vi "Gauss-fit_smpl.vi"(5 "parameter bounds":T2, 6 "initial guess":T1, 10 "FF array":dbl[](array[numeric])=[275.0, 9.0, -4.0, 1.0, -14.0, 8.0, 1.0, 17.0, -3.0, 12.0, 6.0, 9.0, -11.0, -4.0, -2.0, 0.0, -2.0, -7.0, 7.0, -2.0, -2.0, -13.0, 2.0, -1.0, -16.0, 3.0, -2.0, -3.0, 2.0, -2.0, 1.0, -1.0, -15.0, -12.0, -11.0, -10.0, -8.0, 13.0, -3.0, 3.0, 10.0, 2.0, -4.0, 2.0, 5.0, 9.0, 20.0, 3.0, -2.0, 9.0, -1.0, 9.0, -8.0, 11.0, 8.0, 19.0, 1.0, -1.0, -1.0, -9.0, -4.0, -5.0, -2.0, -4.0, -16.0, -10.0, -11.0, -12.0, -4.0, -3.0, -10.0, -5.0, -6.0, -8.0, 10.0, 11.0, -9.0, 2.0, 5.0, 6.0, -7.0, 1.0, 2.0, -2.0, -4.0, -10.0, -8.0, 2.0, -3.0, -7.0, 5.0, 5.0, -8.0, 2.0, -3.0, 19.0, -1.0, 9.0, 10.0, 19.0, 10.0, 9.0, 14.0, 8.0, 0.0, 6.0, 5.0, 3.0, -10.0, -7.0, 0.0, -12.0, -21.0, -3.0, -14.0, 5.0, -4.0, 2.0, -2.0, 0.0, -8.0, 12.0, 1.0, -5.0, -10.0, -8.0, -4.0, -12.0, 1.0, -12.0, -7.0, 7.0, 5.0, 7.0, -3.0, 13.0, 16.0, 13.0, -16.0, 25.0, 7.0, -1.0, 1.0, 20.0, 16.0, 7.0, 9.0, 13.0, 7.0, 10.0, 5.0, 6.0, -1.0, -1.0, -2.0, -10.0, -15.0, -8.0, -27.0, -5.0, -7.0, 5.0, 2.0, 15.0, 3.0, 0.0, 8.0, -1.0, 1.0, 3.0, -6.0, 0.0, 3.0, 0.0, -12.0, 7.0, -7.0, -3.0, 3.0, 2.0, 0.0, -12.0, 4.0, -3.0, -7.0, 6.0, -11.0, 6.0, 0.0, -3.0, -4.0, 1.0, 1.0, 4.0, -6.0, 14.0, 3.0, 7.0, 5.0, 4.0, 2.0, 4.0, 13.0, 0.0, 6.0, -12.0, 0.0, 2.0, -9.0, -4.0, 9.0, 11.0, -2.0, 10.0, 1.0, 4.0, 14.0, 3.0, -1.0, 19.0, 12.0, -12.0, 7.0, -14.0, -5.0, 1.0, -1.0, -8.0, -2.0, -7.0, 0.0, -2.0, 5.0, -8.0, -2.0, 14.0, -6.0, 6.0, 5.0, 4.0, 5.0, -3.0, -8.0, -9.0, -15.0, 8.0, -2.0, 3.0, -3.0, 12.0, 4.0, 9.0, 1.0, 10.0, 4.0, 6.0, 0.0, -13.0, -15.0, -8.0, -9.0, -8.0, -6.0, -20.0, -3.0, -6.0, -8.0, 1.0, -7.0, -17.0, -4.0, 2.0, -17.0, 1.0, -2.0, 4.0, 4.0, 14.0, -1.0, 5.0, -1.0, 7.0, -3.0, -2.0, 5.0, -1.0, 8.0, 11.0, 15.0, 3.0, 12.0, 20.0, 5.0, 13.0, 6.0, 22.0, 1.0, 4.0, 7.0, 15.0, 4.0, -1.0, 13.0, 11.0, 6.0, 3.0, 8.0, -2.0, -3.0, 9.0, 15.0, 5.0, 16.0, 5.0, 2.0, 5.0, -5.0, 5.0, -7.0, -8.0, -8.0, -11.0, -13.0, -1.0, -12.0, 6.0, -2.0, 11.0, -2.0, 2.0, -12.0, -10.0, -13.0, -4.0, -13.0, -9.0, 8.0, -5.0, -7.0, -8.0, -8.0, 1.0, -1.0, 4.0, 12.0, 3.0, 8.0, 2.0, 3.0, 6.0, -12.0, 12.0, 5.0, 4.0, 2.0, -10.0, 3.0, -9.0, 8.0, 16.0, -6.0, 7.0, -2.0, 15.0, 7.0, 12.0, -1.0, 19.0, 5.0, -17.0, -8.0, -1.0, -15.0, 2.0, -11.0, 1.0, 2.0, 0.0, 3.0, -13.0, -3.0, -3.0, 11.0, 12.0, 7.0, 26.0, 5.0, 22.0, 9.0, 17.0, 2.0, 5.0, 13.0, 5.0, 8.0, 0.0, 0.0, -11.0, 16.0, 18.0, 0.0, 24.0, 6.0, 20.0, 9.0, 6.0, 7.0, 14.0, 4.0, 2.0, -4.0, 15.0, 7.0, 4.0, 4.0, -3.0, -3.0, 4.0, 4.0, -3.0, -3.0, 6.0, 8.0, 11.0, 3.0, 9.0, 0.0, 18.0, -5.0, 0.0, 3.0, -9.0, -1.0, -5.0, 3.0, 1.0, -16.0, -4.0, -4.0, -1.0, -3.0, 1.0, 5.0, -12.0, -11.0, -2.0, -16.0, -2.0, -23.0, 18.0, 1.0, 24.0, -3.0, 10.0, 3.0, 4.0, -2.0, 7.0, 0.0, 7.0, -2.0, -4.0, 7.0, 4.0, 11.0, 13.0, 14.0, 8.0, 3.0, -2.0, -1.0, 7.0, -9.0, -13.0, 0.0, 1.0, 6.0, -4.0, -7.0, 2.0, -4.0, -1.0, -7.0, 11.0, -7.0, -5.0, -7.0, -8.0, -9.0, -9.0, -5.0, 4.0, -10.0, -8.0, 5.0, -8.0, 2.0, 4.0, 6.0, 0.0, 3.0, -3.0, 4.0, -4.0, -8.0, -1.0, -1.0, -1.0, -7.0, -19.0, 8.0, 0.0, 0.0, -11.0, -10.0, -11.0, -9.0, -7.0, -15.0, -9.0, -5.0, -1.0, 2.0, -3.0, -6.0, 0.0, 2.0, -7.0, -9.0, -8.0, 1.0, -2.0, 0.0, -7.0, -12.0, 10.0, 3.0, -4.0, -8.0, -7.0, 6.0, -5.0, 9.0, -11.0, 11.0, -13.0, -6.0, 1.0, -1.0, 1.0, -8.0, -5.0, -8.0, -5.0, -5.0, 2.0, 13.0, 13.0, 1.0, 6.0, -1.0, 15.0, -8.0, -5.0, 0.0, 0.0, 9.0, -2.0, 2.0, 2.0, 7.0, -8.0, 10.0, 2.0, -15.0, -17.0, 5.0, -16.0, -8.0, -12.0, -2.0, -13.0, 1.0, -9.0, -5.0, -7.0, -6.0, -10.0, -3.0, -12.0, -6.0, -8.0, -14.0, 3.0, -6.0, -2.0, 2.0, 0.0, -1.0, 6.0, 6.0, 1.0, -5.0, 2.0, -6.0, -12.0, -4.0, -4.0, 9.0, 4.0, -2.0, -5.0, 9.0, 3.0, 10.0, 7.0, 7.0, 5.0, 1.0, 5.0, 13.0, 6.0, 14.0, 11.0, 9.0, 14.0, -12.0, -3.0, 8.0, 13.0, -3.0, 7.0, 1.0, 13.0, 11.0, 12.0, 17.0, 7.0, 14.0, 2.0, -1.0, 10.0, -2.0, -3.0, -3.0, -6.0, 8.0, -14.0, 0.0, -2.0, -1.0, -11.0, -4.0, -9.0, -23.0, -4.0, 10.0, -7.0, 8.0, -2.0, 7.0, 0.0, -5.0, 0.0, 11.0, 2.0, 1.0, -1.0, -12.0, -3.0, 4.0, -4.0, 5.0, -9.0, 9.0, 5.0, 4.0, -7.0, 2.0, 5.0, -2.0, -9.0, -2.0, -13.0, 2.0, -5.0, -15.0, -3.0, -13.0, -4.0, -9.0, -14.0, -4.0, 6.0, 9.0, -1.0, 2.0, -8.0, -4.0, -4.0, -5.0, -19.0, -19.0, -7.0, -7.0, 1.0, -6.0, -4.0, 9.0, -6.0, 6.0, 14.0, 12.0, 4.0, 11.0, 3.0, -1.0, 14.0, 12.0, -3.0, 15.0, 6.0, 9.0, 5.0, 2.0, 5.0, 6.0, -4.0, 16.0, 12.0, 22.0, 4.0, 14.0, 1.0, 9.0, 10.0, 12.0, 6.0, 5.0, 1.0, 4.0, -6.0, 3.0, -10.0, 3.0, -5.0, 8.0, 13.0, -1.0, -4.0, -7.0, -12.0, 6.0, -14.0, -17.0, -13.0, -9.0, -11.0, -16.0, -11.0, -8.0, -14.0, -20.0, -10.0, -15.0, -9.0, -8.0, -13.0, 5.0, -7.0, 5.0, 0.0, -6.0, 9.0, 12.0, -4.0, -13.0, -1.0, -8.0, -15.0, -13.0, -25.0, -8.0, -16.0, -9.0, 3.0, 5.0, -9.0, -1.0, 3.0, 5.0, -2.0, 15.0, -5.0, -8.0, -8.0, -15.0, 0.0, -13.0, -10.0, -9.0, 1.0, -6.0, 2.0, 0.0, -9.0, 8.0, -2.0, -1.0, -5.0, 6.0, -3.0, 5.0, 7.0, -1.0, -3.0, 1.0, 2.0, -18.0, 10.0, 9.0, 23.0, 8.0, 14.0, -3.0, 9.0, -1.0, 5.0, -18.0, -8.0, -7.0, -4.0, 6.0, -14.0, -1.0, -2.0, -4.0, -8.0, -2.0, -11.0, 3.0, -2.0, 0.0, -4.0, 1.0, -12.0, -1.0, -6.0, 4.0, -16.0, -1.0, -1.0, -8.0, -9.0, 5.0, -7.0, -6.0, -1.0, 13.0, 1.0, 3.0, -13.0, 4.0, -5.0, 9.0, -13.0, -3.0, -15.0, -27.0, -10.0, -7.0, 3.0, 0.0, 1.0, 13.0, -3.0, 5.0, -3.0, 14.0, 2.0, -3.0, -4.0, 1.0, 4.0, 4.0, -6.0, 16.0, 8.0, 20.0, 11.0, 0.0, 6.0, 7.0, -1.0, -16.0, -8.0, 0.0, -9.0, -9.0, -12.0, 8.0, -9.0, 2.0, -13.0, -4.0, -4.0, -8.0, -20.0, 2.0, -13.0, -7.0, -8.0, -2.0, -6.0, -3.0, -15.0, -13.0, 6.0, -6.0, -1.0, 18.0, 7.0, 14.0, 2.0, 6.0, 10.0, 3.0, 0.0, 13.0, -8.0, -2.0, 0.0, -2.0, 12.0, -18.0, -1.0, 0.0, -25.0, -1.0, -4.0, 2.0, 2.0, -4.0, -7.0, 6.0, 4.0, 4.0, -2.0, 12.0, 14.0, -7.0, 4.0, -13.0, -5.0, -7.0, -6.0, -12.0, -3.0, -18.0, -16.0, -3.0, 2.0, -9.0, -2.0, -7.0, 1.0, 14.0, -15.0, 16.0, -2.0, -4.0, 2.0, 14.0, -4.0, 1.0, 1.0, 2.0, -7.0, -8.0, 5.0, -2.0, -4.0, 1.0, 3.0, -1.0, -4.0, 1.0, -6.0, -2.0, -7.0, -3.0, -12.0, -1.0, -14.0, -15.0, -6.0, -4.0, -5.0, -9.0, -15.0, -5.0, -10.0, -4.0, -18.0, 10.0, 2.0, -6.0, -2.0, -1.0, -6.0, -10.0, -6.0, 1.0, 7.0, -4.0, -1.0, 12.0, 2.0, 1.0, -6.0, 7.0, -22.0, 4.0, 267.0] format="%.4f") -> (0 "standard deviation":dbl, 1 "center":dbl, 2 "amplitude":dbl, 3 "Best fit array":dbl[](array[numeric])=[275.0, 9.0, -4.0, 1.0, -14.0, 8.0, 1.0, 17.0, -3.0, 12.0, 6.0, 9.0, -11.0, -4.0, -2.0, 0.0, -2.0, -7.0, 7.0, -2.0, -2.0, -13.0, 2.0, -1.0, -16.0, 3.0, -2.0, -3.0, 2.0, -2.0, 1.0, -1.0, -15.0, -12.0, -11.0, -10.0, -8.0, 13.0, -3.0, 3.0, 10.0, 2.0, -4.0, 2.0, 5.0, 9.0, 20.0, 3.0, -2.0, 9.0, -1.0, 9.0, -8.0, 11.0, 8.0, 19.0, 1.0, -1.0, -1.0, -9.0, -4.0, -5.0, -2.0, -4.0, -16.0, -10.0, -11.0, -12.0, -4.0, -3.0, -10.0, -5.0, -6.0, -8.0, 10.0, 11.0, -9.0, 2.0, 5.0, 6.0, -7.0, 1.0, 2.0, -2.0, -4.0, -10.0, -8.0, 2.0, -3.0, -7.0, 5.0, 5.0, -8.0, 2.0, -3.0, 19.0, -1.0, 9.0, 10.0, 19.0, 10.0, 9.0, 14.0, 8.0, 0.0, 6.0, 5.0, 3.0, -10.0, -7.0, 0.0, -12.0, -21.0, -3.0, -14.0, 5.0, -4.0, 2.0, -2.0, 0.0, -8.0, 12.0, 1.0, -5.0, -10.0, -8.0, -4.0, -12.0, 1.0, -12.0, -7.0, 7.0, 5.0, 7.0, -3.0, 13.0, 16.0, 13.0, -16.0, 25.0, 7.0, -1.0, 1.0, 20.0, 16.0, 7.0, 9.0, 13.0, 7.0, 10.0, 5.0, 6.0, -1.0, -1.0, -2.0, -10.0, -15.0, -8.0, -27.0, -5.0, -7.0, 5.0, 2.0, 15.0, 3.0, 0.0, 8.0, -1.0, 1.0, 3.0, -6.0, 0.0, 3.0, 0.0, -12.0, 7.0, -7.0, -3.0, 3.0, 2.0, 0.0, -12.0, 4.0, -3.0, -7.0, 6.0, -11.0, 6.0, 0.0, -3.0, -4.0, 1.0, 1.0, 4.0, -6.0, 14.0, 3.0, 7.0, 5.0, 4.0, 2.0, 4.0, 13.0, 0.0, 6.0, -12.0, 0.0, 2.0, -9.0, -4.0, 9.0, 11.0, -2.0, 10.0, 1.0, 4.0, 14.0, 3.0, -1.0, 19.0, 12.0, -12.0, 7.0, -14.0, -5.0, 1.0, -1.0, -8.0, -2.0, -7.0, 0.0, -2.0, 5.0, -8.0, -2.0, 14.0, -6.0, 6.0, 5.0, 4.0, 5.0, -3.0, -8.0, -9.0, -15.0, 8.0, -2.0, 3.0, -3.0, 12.0, 4.0, 9.0, 1.0, 10.0, 4.0, 6.0, 0.0, -13.0, -15.0, -8.0, -9.0, -8.0, -6.0, -20.0, -3.0, -6.0, -8.0, 1.0, -7.0, -17.0, -4.0, 2.0, -17.0, 1.0, -2.0, 4.0, 4.0, 14.0, -1.0, 5.0, -1.0, 7.0, -3.0, -2.0, 5.0, -1.0, 8.0, 11.0, 15.0, 3.0, 12.0, 20.0, 5.0, 13.0, 6.0, 22.0, 1.0, 4.0, 7.0, 15.0, 4.0, -1.0, 13.0, 11.0, 6.0, 3.0, 8.0, -2.0, -3.0, 9.0, 15.0, 5.0, 16.0, 5.0, 2.0, 5.0, -5.0, 5.0, -7.0, -8.0, -8.0, -11.0, -13.0, -1.0, -12.0, 6.0, -2.0, 11.0, -2.0, 2.0, -12.0, -10.0, -13.0, -4.0, -13.0, -9.0, 8.0, -5.0, -7.0, -8.0, -8.0, 1.0, -1.0, 4.0, 12.0, 3.0, 8.0, 2.0, 3.0, 6.0, -12.0, 12.0, 5.0, 4.0, 2.0, -10.0, 3.0, -9.0, 8.0, 16.0, -6.0, 7.0, -2.0, 15.0, 7.0, 12.0, -1.0, 19.0, 5.0, -17.0, -8.0, -1.0, -15.0, 2.0, -11.0, 1.0, 2.0, 0.0, 3.0, -13.0, -3.0, -3.0, 11.0, 12.0, 7.0, 26.0, 5.0, 22.0, 9.0, 17.0, 2.0, 5.0, 13.0, 5.0, 8.0, 0.0, 0.0, -11.0, 16.0, 18.0, 0.0, 24.0, 6.0, 20.0, 9.0, 6.0, 7.0, 14.0, 4.0, 2.0, -4.0, 15.0, 7.0, 4.0, 4.0, -3.0, -3.0, 4.0, 4.0, -3.0, -3.0, 6.0, 8.0, 11.0, 3.0, 9.0, 0.0, 18.0, -5.0, 0.0, 3.0, -9.0, -1.0, -5.0, 3.0, 1.0, -16.0, -4.0, -4.0, -1.0, -3.0, 1.0, 5.0, -12.0, -11.0, -2.0, -16.0, -2.0, -23.0, 18.0, 1.0, 24.0, -3.0, 10.0, 3.0, 4.0, -2.0, 7.0, 0.0, 7.0, -2.0, -4.0, 7.0, 4.0, 11.0, 13.0, 14.0, 8.0, 3.0, -2.0, -1.0, 7.0, -9.0, -13.0, 0.0, 1.0, 6.0, -4.0, -7.0, 2.0, -4.0, -1.0, -7.0, 11.0, -7.0, -5.0, -7.0, -8.0, -9.0, -9.0, -5.0, 4.0, -10.0, -8.0, 5.0, -8.0, 2.0, 4.0, 6.0, 0.0, 3.0, -3.0, 4.0, -4.0, -8.0, -1.0, -1.0, -1.0, -7.0, -19.0, 8.0, 0.0, 0.0, -11.0, -10.0, -11.0, -9.0, -7.0, -15.0, -9.0, -5.0, -1.0, 2.0, -3.0, -6.0, 0.0, 2.0, -7.0, -9.0, -8.0, 1.0, -2.0, 0.0, -7.0, -12.0, 10.0, 3.0, -4.0, -8.0, -7.0, 6.0, -5.0, 9.0, -11.0, 11.0, -13.0, -6.0, 1.0, -1.0, 1.0, -8.0, -5.0, -8.0, -5.0, -5.0, 2.0, 13.0, 13.0, 1.0, 6.0, -1.0, 15.0, -8.0, -5.0, 0.0, 0.0, 9.0, -2.0, 2.0, 2.0, 7.0, -8.0, 10.0, 2.0, -15.0, -17.0, 5.0, -16.0, -8.0, -12.0, -2.0, -13.0, 1.0, -9.0, -5.0, -7.0, -6.0, -10.0, -3.0, -12.0, -6.0, -8.0, -14.0, 3.0, -6.0, -2.0, 2.0, 0.0, -1.0, 6.0, 6.0, 1.0, -5.0, 2.0, -6.0, -12.0, -4.0, -4.0, 9.0, 4.0, -2.0, -5.0, 9.0, 3.0, 10.0, 7.0, 7.0, 5.0, 1.0, 5.0, 13.0, 6.0, 14.0, 11.0, 9.0, 14.0, -12.0, -3.0, 8.0, 13.0, -3.0, 7.0, 1.0, 13.0, 11.0, 12.0, 17.0, 7.0, 14.0, 2.0, -1.0, 10.0, -2.0, -3.0, -3.0, -6.0, 8.0, -14.0, 0.0, -2.0, -1.0, -11.0, -4.0, -9.0, -23.0, -4.0, 10.0, -7.0, 8.0, -2.0, 7.0, 0.0, -5.0, 0.0, 11.0, 2.0, 1.0, -1.0, -12.0, -3.0, 4.0, -4.0, 5.0, -9.0, 9.0, 5.0, 4.0, -7.0, 2.0, 5.0, -2.0, -9.0, -2.0, -13.0, 2.0, -5.0, -15.0, -3.0, -13.0, -4.0, -9.0, -14.0, -4.0, 6.0, 9.0, -1.0, 2.0, -8.0, -4.0, -4.0, -5.0, -19.0, -19.0, -7.0, -7.0, 1.0, -6.0, -4.0, 9.0, -6.0, 6.0, 14.0, 12.0, 4.0, 11.0, 3.0, -1.0, 14.0, 12.0, -3.0, 15.0, 6.0, 9.0, 5.0, 2.0, 5.0, 6.0, -4.0, 16.0, 12.0, 22.0, 4.0, 14.0, 1.0, 9.0, 10.0, 12.0, 6.0, 5.0, 1.0, 4.0, -6.0, 3.0, -10.0, 3.0, -5.0, 8.0, 13.0, -1.0, -4.0, -7.0, -12.0, 6.0, -14.0, -17.0, -13.0, -9.0, -11.0, -16.0, -11.0, -8.0, -14.0, -20.0, -10.0, -15.0, -9.0, -8.0, -13.0, 5.0, -7.0, 5.0, 0.0, -6.0, 9.0, 12.0, -4.0, -13.0, -1.0, -8.0, -15.0, -13.0, -25.0, -8.0, -16.0, -9.0, 3.0, 5.0, -9.0, -1.0, 3.0, 5.0, -2.0, 15.0, -5.0, -8.0, -8.0, -15.0, 0.0, -13.0, -10.0, -9.0, 1.0, -6.0, 2.0, 0.0, -9.0, 8.0, -2.0, -1.0, -5.0, 6.0, -3.0, 5.0, 7.0, -1.0, -3.0, 1.0, 2.0, -18.0, 10.0, 9.0, 23.0, 8.0, 14.0, -3.0, 9.0, -1.0, 5.0, -18.0, -8.0, -7.0, -4.0, 6.0, -14.0, -1.0, -2.0, -4.0, -8.0, -2.0, -11.0, 3.0, -2.0, 0.0, -4.0, 1.0, -12.0, -1.0, -6.0, 4.0, -16.0, -1.0, -1.0, -8.0, -9.0, 5.0, -7.0, -6.0, -1.0, 13.0, 1.0, 3.0, -13.0, 4.0, -5.0, 9.0, -13.0, -3.0, -15.0, -27.0, -10.0, -7.0, 3.0, 0.0, 1.0, 13.0, -3.0, 5.0, -3.0, 14.0, 2.0, -3.0, -4.0, 1.0, 4.0, 4.0, -6.0, 16.0, 8.0, 20.0, 11.0, 0.0, 6.0, 7.0, -1.0, -16.0, -8.0, 0.0, -9.0, -9.0, -12.0, 8.0, -9.0, 2.0, -13.0, -4.0, -4.0, -8.0, -20.0, 2.0, -13.0, -7.0, -8.0, -2.0, -6.0, -3.0, -15.0, -13.0, 6.0, -6.0, -1.0, 18.0, 7.0, 14.0, 2.0, 6.0, 10.0, 3.0, 0.0, 13.0, -8.0, -2.0, 0.0, -2.0, 12.0, -18.0, -1.0, 0.0, -25.0, -1.0, -4.0, 2.0, 2.0, -4.0, -7.0, 6.0, 4.0, 4.0, -2.0, 12.0, 14.0, -7.0, 4.0, -13.0, -5.0, -7.0, -6.0, -12.0, -3.0, -18.0, -16.0, -3.0, 2.0, -9.0, -2.0, -7.0, 1.0, 14.0, -15.0, 16.0, -2.0, -4.0, 2.0, 14.0, -4.0, 1.0, 1.0, 2.0, -7.0, -8.0, 5.0, -2.0, -4.0, 1.0, 3.0, -1.0, -4.0, 1.0, -6.0, -2.0, -7.0, -3.0, -12.0, -1.0, -14.0, -15.0, -6.0, -4.0, -5.0, -9.0, -15.0, -5.0, -10.0, -4.0, -18.0, 10.0, 2.0, -6.0, -2.0, -1.0, -6.0, -10.0, -6.0, 1.0, 7.0, -4.0, -1.0, 12.0, 2.0, 1.0, -6.0, 7.0, -22.0, 4.0, 267.0] format="%.4f", 4 "initial guess ADJ":T1)   [LabVIEW 2016]
uses:
  <vilib>/Analysis/baseanly.llb/Mean (DBL).vi
  <vilib>/Analysis/NI_AALPro.lvlib
  <vilib>/Analysis/NI_AALBase.lvlib
panel:
  out "Slice 3":dbl[][](graph)
  out "median":dbl format="%0.2f"
  out "mean":dbl format="%0.2f"
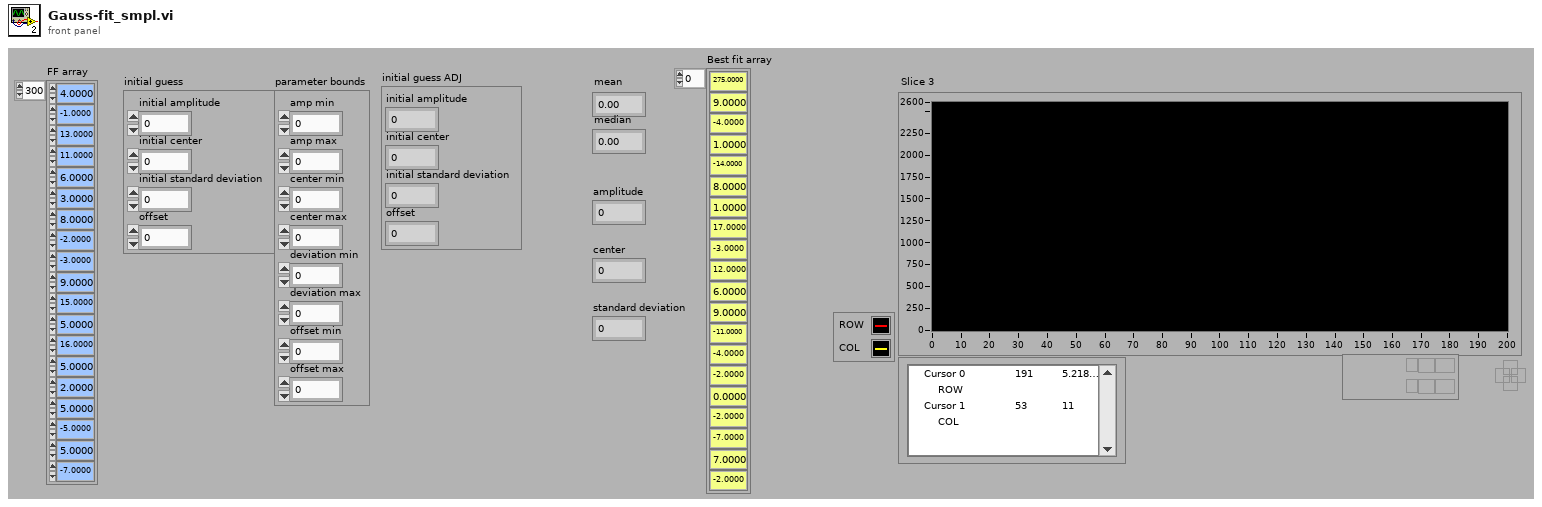
[diagram p1: front panel]
types:
  T1 = cluster{"initial amplitude":dbl, "initial center":dbl, "initial standard deviation":dbl, "offset":dbl}
  T2 = cluster{"amp min":dbl, "amp max":dbl, "center min":dbl, "center max":dbl, "deviation min":dbl, "deviation max":dbl, "offset min":dbl, "offset max":dbl}
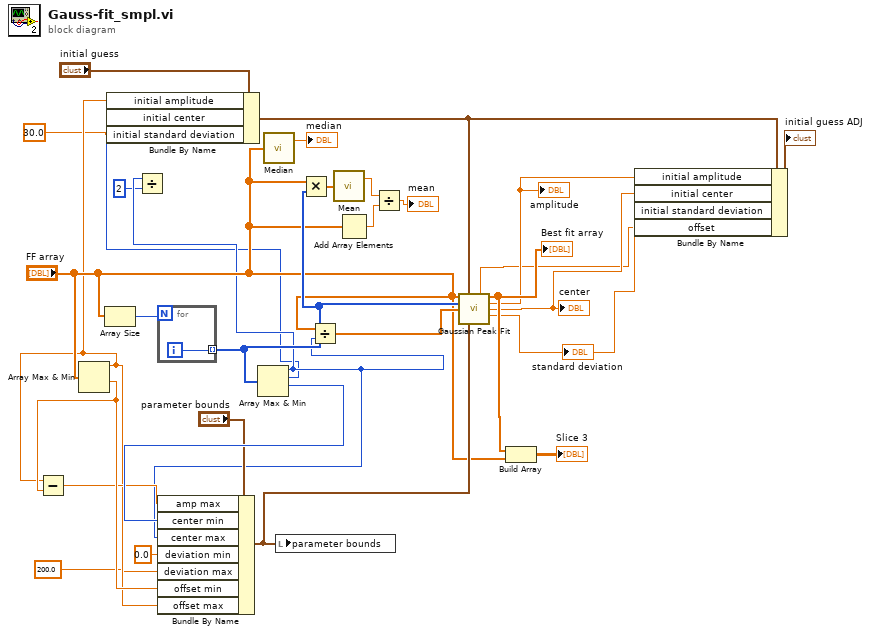
[diagram p0: block diagram]
diagram:
  n1 = Array Max & Min(array="FF array") -> (max value=w12:dbl, min value=w20:dbl)  [unwired: 2 out]
  n2 = Subtract(x=w12, y=w20) -> (x-y=w19:dbl)
  n3 = Array Size(array="FF array") -> (size(s)=w24:i32)
  n4 = for {
    N: w24 -> [_]
    tunnel: [w31] -> w22 mode=indexing
    i -> [w31]
  }
  n5 = Array Max & Min(array=w22) -> (max value=w11:i32, max index (indices)=w7:i32, min value=w23:i32)  [unwired: 1 out]
  n6 = Bundle By Name(cluster="initial guess", "initial amplitude"=w12, "initial center"=w7, "initial standard deviation"=30.0) -> (w6:T1)
  n7 = Divide(x=w11, y=2) -> ()  [unwired: 1 out]
  n8 = Bundle By Name(cluster="parameter bounds", "amp max"=w19, "center min"=w23, "center max"=w11, "deviation min"=0.0, "deviation max"=200.0 ("deviation min"), "offset min"=w20, "offset max"=w12) -> (w18:T2)
  n9 = call <vilib>:"Median.vi"("X"="FF array") -> ("median"=→"median":dbl)  [unwired: 1 out]
  n10 = local write "parameter bounds"(w18) -> ()
  n11 = Multiply(x="FF array", y=w22) -> (x*y=w29:dbl[])
  n12 = Divide(x="FF array", y=w11) -> (x/y=w30:dbl[])
  n13 = call-poly <vilib>:"Mean.vi"("X"=w29) -> ("mean"=w25:dbl)  [unwired: 1 out]
  n14 = Add Array Elements(numeric array="FF array") -> (sum=w27:dbl)
  n15 = Divide(x=w25, y=w27) -> (x/y=→"mean":dbl)
  n16 = call <vilib>:"Gaussian Peak Fit.vi"("Y"="FF array", "initial guess"=w6, "X"=w22, "Weight"=w30, "parameter bounds"=w18) -> ("offset"=w2:dbl, "Best Gaussian Fit"=w16:dbl[], "amplitude"=w5:dbl, "center"=w4:dbl, "standard deviation"=w3:dbl)  [unwired: 4 in, 2 out]
  "standard deviation" <- w3
  "center" <- w4
  "amplitude" <- w5
  "Best fit array" <- w16
  n17 = Build Array(w16, "FF array") -> (→"Slice 3":dbl[][])
  n18 = Bundle By Name(cluster=w6, "initial amplitude"=w5, "initial center"=w4, "initial standard deviation"=w3, "offset"=w2) -> (→"initial guess ADJ":T1)
